vi "Identify - ModuleScan.vi"(8 "Fehler (Eingang, kein Fehler)":errorcluster) -> (0 "Fehler (Ausgang)":errorcluster, 3 "LifeList":T1(array[cluster]))   [LabVIEW 2016]
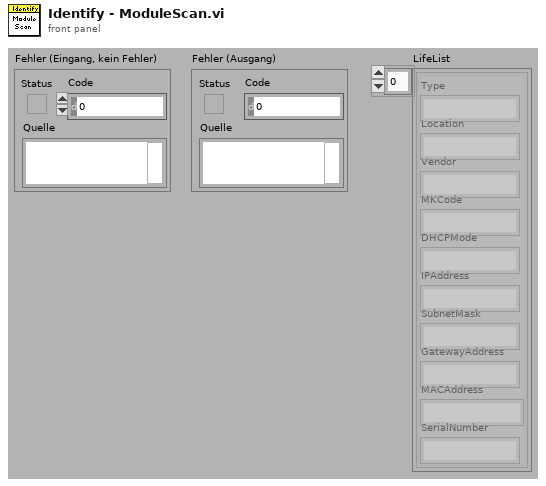
[diagram p1: front panel]
types:
  T1 = cluster{"Type":string, "Location":string, "Vendor":string, "MKCode":string, "DHCPMode":string, "IPAddress":string, "SubnetMask":string, "GatewayAddress":string, "MACAddress":string, "SerialNumber":string}[]
  T2 = cluster{"Type":string, "Location":string, "Vendor":string, "MKCode":string, "DHCPMode":string, "IPAddress":string, "SubnetMask":string, "GatewayAddress":string, "MACAddress":string, "SerialNumber":string}
  T3 = cluster{"HighSpeedPort":path, "Utility":path, "Ismbus32":path}
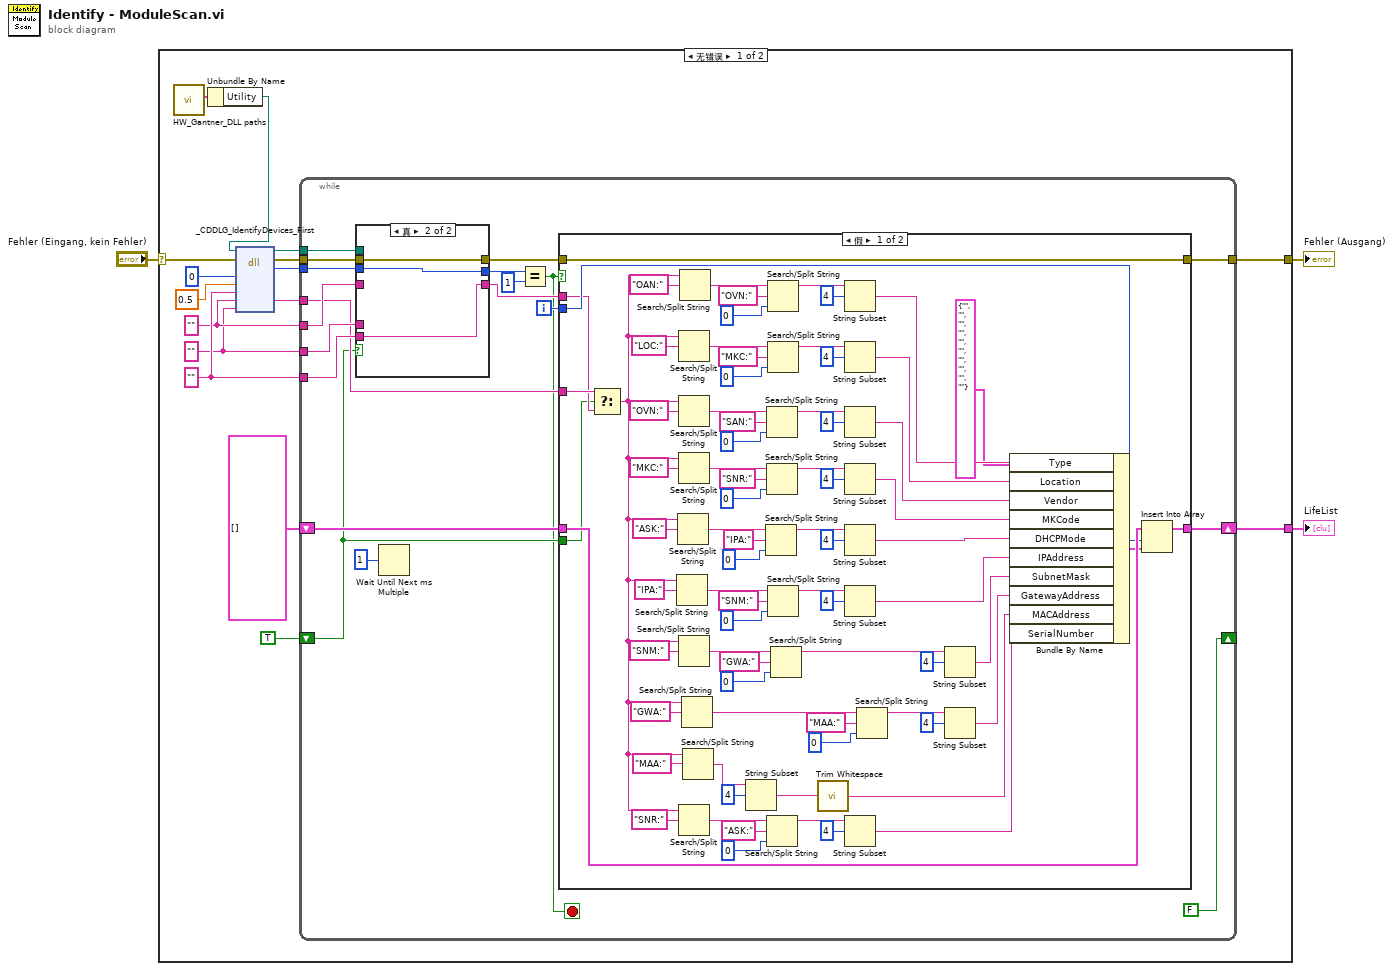
[diagram p0: block diagram]
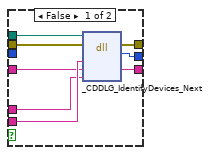
[diagram p3: hidden frame]
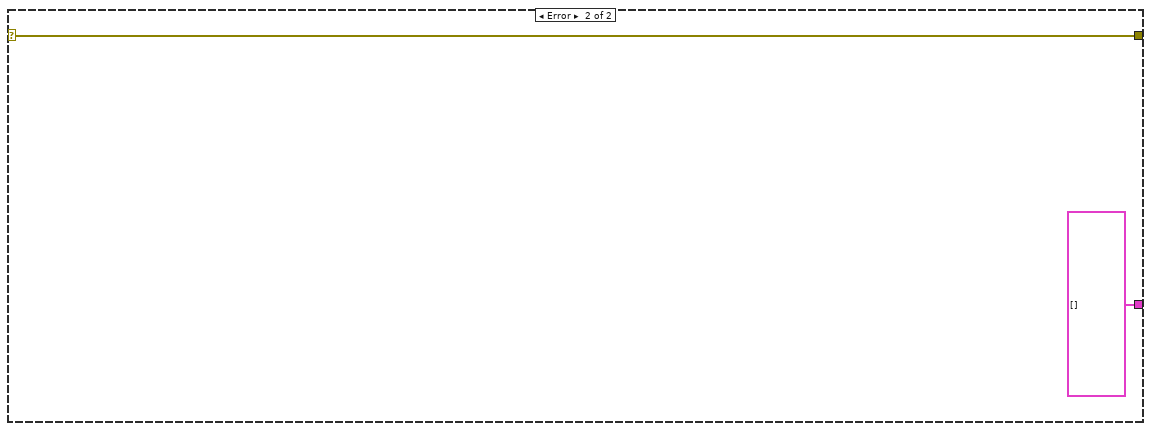
[diagram p4: hidden frame]
diagram:
  n1 = case shown="无错误" "Fehler (Eingang, kein Fehler)" {
    selector: "Fehler (Eingang, kein Fehler)" -> [w8 w131]
    tunnel: [w7 w131] -> w1
    tunnel: [w19 T1 []] -> w2
    frame No Error {
      w14 = "" ("ErrorString")
      w15 = "" ("DeviceInfo")
      w16 = "" ("AdapterInfo")
      n2 = call "HW_Gantner_DLL paths.vi"() -> ("DLL paths"=w6:T3)  [unwired: 11 in]
      n3 = Unbundle By Name(w6) -> ("Utility"=w4:path)
      n4 = dll-call lib="eGateUtility.dll" fn="_CDDLG_IdentifyDevices_First"(path in=w4, error in=w8, "ExtCommand"=0, "ScanTime"=0.5, "AdapterInfo"=w16, "DeviceInfo"=w15, "ErrorString"=w14) -> (path out=w5:path, error out=w9:errorcluster, "Rückgabetyp"=w10:i32, "DeviceInfo"=w13:string)  [unwired: 3 in, 2 out]
      n5 = while {
        tunnel: w9 -> [w38]
        tunnel: w16 -> [w37]
        tunnel: w15 -> [w36]
        tunnel: w14 -> [w35]
        shift-right: [w32] -> w19
        shift-left: T1 [] -> [w34]
        tunnel: w13 -> [w30]
        shift-right: [FALSE] -> _
        shift-left: TRUE -> [w28]
        tunnel: w10 -> [w24]
        tunnel: [w23] -> w7
        tunnel: w5 -> [w20]
        i -> [w33]
        stop <- w22 stop-if-true
        n6 = case shown="真" w28 {
          tunnel: w38 -> [w126 w127]
          tunnel: w37 -> [w125 w128]
          tunnel: w36 -> [w124 _]
          tunnel: w35 -> [w123 _]
          tunnel: [w122 w129] -> w25
          tunnel: [w121 w127] -> w31
          tunnel: [w120 w128] -> w29
          tunnel: w24 -> [_ w129]
          tunnel: w20 -> [w119 _]
          frame False {
            n7 = dll-call lib="eGateUtility.dll" fn="_CDDLG_IdentifyDevices_Next"(path in=w119, error in=w126, "AdapterInfo"=w125, "DeviceInfo"=w124, "ErrorString"=w123) -> (error out=w121:errorcluster, "Rückgabetyp"=w122:i32, "DeviceInfo"=w120:string)  [unwired: 1 in, 3 out]
          }
          frame True {
          }
        }
        n8 = Wait Until Next ms Multiple(millisecond multiple=u32 1 ("Vielfache von ms")) -> ()  [unwired: 1 out]
        n9 = Equal?(x=w25, y=1) -> (x = y?=w22:bool)
        n10 = case shown="假" w22 {
          tunnel: w34 -> [w116 w118]
          tunnel: w33 -> [w115 _]
          tunnel: [w114 w118] -> w32
          tunnel: w31 -> [w98 w117]
          tunnel: [w98 w117] -> w23
          tunnel: w30 -> [w101 _]
          tunnel: w29 -> [w100 _]
          tunnel: w28 -> [w99 _]
          frame False {
            n11 = Select(t=w101, s=w99, f=w100) -> (s? t:f=w42:string)
            n12 = Search/Split String(string=w42, search string/char (-)="IPA:" ("Nach String/Zeichen suchen (-)")) -> (match + rest of string=w111:string)  [unwired: 3 out]
            n13 = Search/Split String(string=w42, search string/char (-)="ASK:" ("Nach String/Zeichen suchen (-)")) -> (match + rest of string=w70:string)  [unwired: 3 out]
            n14 = Search/Split String(string=w42, search string/char (-)="LOC:" ("Nach String/Zeichen suchen (-)")) -> (match + rest of string=w107:string)  [unwired: 3 out]
            n15 = Search/Split String(string=w42, search string/char (-)="OVN:" ("Nach String/Zeichen suchen (-)")) -> (match + rest of string=w88:string)  [unwired: 3 out]
            n16 = Search/Split String(string=w42, search string/char (-)="MKC:" ("Nach String/Zeichen suchen (-)")) -> (match + rest of string=w82:string)  [unwired: 3 out]
            n17 = Search/Split String(string=w42, search string/char (-)="SNM:" ("Nach String/Zeichen suchen (-)")) -> (match + rest of string=w64:string)  [unwired: 3 out]
            n18 = Search/Split String(string=w42, search string/char (-)="SNR:" ("Nach String/Zeichen suchen (-)")) -> (match + rest of string=w76:string)  [unwired: 3 out]
            n19 = Search/Split String(string=w42, search string/char (-)="OAN:" ("Nach String/Zeichen suchen (-)")) -> (match + rest of string=w94:string)  [unwired: 3 out]
            n20 = Search/Split String(string=w42, search string/char (-)="GWA:" ("Nach String/Zeichen suchen (-)")) -> (match + rest of string=w50:string)  [unwired: 3 out]
            n21 = Search/Split String(string=w42, search string/char (-)="MAA:" ("Nach String/Zeichen suchen (-)")) -> (match + rest of string=w41:string)  [unwired: 3 out]
            n22 = String Subset(string=w41, offset (0)=4 ("Offset (0)")) -> (substring=w40:string)  [unwired: 1 out]
            n23 = Search/Split String(string=w70, search string/char (-)="IPA:" ("Nach String/Zeichen suchen (-)"), offset (0)=0 ("Offset (0)")) -> (substring before match=w68:string)  [unwired: 2 out]
            n24 = Search/Split String(string=w88, search string/char (-)="SAN:" ("Nach String/Zeichen suchen (-)"), offset (0)=0 ("Offset (0)")) -> (substring before match=w86:string)  [unwired: 2 out]
            n25 = Search/Split String(string=w82, search string/char (-)="SNR:" ("Nach String/Zeichen suchen (-)"), offset (0)=0 ("Offset (0)")) -> (substring before match=w80:string)  [unwired: 2 out]
            n26 = Search/Split String(string=w76, search string/char (-)="ASK:" ("Nach String/Zeichen suchen (-)"), offset (0)=0 ("Offset (0)")) -> (substring before match=w74:string)  [unwired: 2 out]
            n27 = Search/Split String(string=w94, search string/char (-)="OVN:" ("Nach String/Zeichen suchen (-)"), offset (0)=0 ("Offset (0)")) -> (substring before match=w92:string)  [unwired: 2 out]
            n28 = Search/Split String(string=w107, search string/char (-)="MKC:" ("Nach String/Zeichen suchen (-)"), offset (0)=0 ("Offset (0)")) -> (substring before match=w105:string)  [unwired: 2 out]
            n29 = Search/Split String(string=w111, search string/char (-)="SNM:" ("Nach String/Zeichen suchen (-)"), offset (0)=0 ("Offset (0)")) -> (substring before match=w104:string)  [unwired: 2 out]
            n30 = Search/Split String(string=w64, search string/char (-)="GWA:" ("Nach String/Zeichen suchen (-)"), offset (0)=0 ("Offset (0)")) -> (substring before match=w62:string)  [unwired: 2 out]
            n31 = call <vilib>:"Trim Whitespace.vi"("string"=w40) -> ("trimmed string"=w39:string)  [unwired: 1 in]
            n32 = String Subset(string=w92, offset (0)=4 ("Offset (0)")) -> (substring=w60:string)  [unwired: 1 out]
            n33 = String Subset(string=w105, offset (0)=4 ("Offset (0)")) -> (substring=w59:string)  [unwired: 1 out]
            n34 = String Subset(string=w86, offset (0)=4 ("Offset (0)")) -> (substring=w57:string)  [unwired: 1 out]
            n35 = String Subset(string=w80, offset (0)=4 ("Offset (0)")) -> (substring=w56:string)  [unwired: 1 out]
            n36 = String Subset(string=w68, offset (0)=4 ("Offset (0)")) -> (substring=w53:string)  [unwired: 1 out]
            n37 = String Subset(string=w104, offset (0)=4 ("Offset (0)")) -> (substring=w58:string)  [unwired: 1 out]
            n38 = String Subset(string=w74, offset (0)=4 ("Offset (0)")) -> (substring=w54:string)  [unwired: 1 out]
            n39 = Search/Split String(string=w50, search string/char (-)="MAA:" ("Nach String/Zeichen suchen (-)"), offset (0)=0 ("Offset (0)")) -> (substring before match=w48:string)  [unwired: 2 out]
            n40 = String Subset(string=w62, offset (0)=4 ("Offset (0)")) -> (substring=w46:string)  [unwired: 1 out]
            n41 = String Subset(string=w48, offset (0)=4 ("Offset (0)")) -> (substring=w45:string)  [unwired: 1 out]
            n42 = Bundle By Name(cluster=T2 {"Type"="", "Location"="", "Vendor"="", "MKCode"="", "DHCPMode"="", "IPAddress"="", "SubnetMask"="", "GatewayAddress"="", "MACAddress"="", "SerialNumber"=""} ("Info"), "Type"=w60, "Location"=w59, "Vendor"=w57, "MKCode"=w56, "DHCPMode"=w53, "IPAddress"=w58, "SubnetMask"=w46, "GatewayAddress"=w45, "MACAddress"=w39, "SerialNumber"=w54) -> (w97:T2)
            n43 = Insert Into Array(array=w116, index=w115, new element=w97) -> (w114:T1)
          }
          frame True {
          }
        }
      }
    }
    frame Error {
    }
  }
  "LifeList" <- w2
  "Fehler (Ausgang)" <- w1
